vi "Sondenmodell.ReadZustandsgrössen.vi"(0 "Sondenmodell in":refnum<data-value>, 5 "error in":errorcluster) -> (14 "Sondenmodell out":refnum<data-value>, 16 "Erdtemperatur [°C]":dbl, 17 "Rücklauftemperatur Solekreislauf [°C]":dbl, 19 "error out":errorcluster)   [LabVIEW 2016, in "Sondenmodell.lvclass"]
uses:
  Sondenmodell.lvclass
  Sondenmodell.lvclass/Sondenmodell.ctl
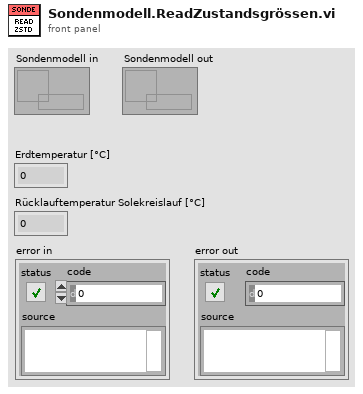
[diagram p1: front panel]
types:
  T1 = typedef "Sondenmodell.lvclass/Sondenmodell.Zustandsgrössen.ctl" = cluster{"Erdtemperatur [°C]":dbl, "Rücklauftemperatur Solekreislauf [°C]":dbl}
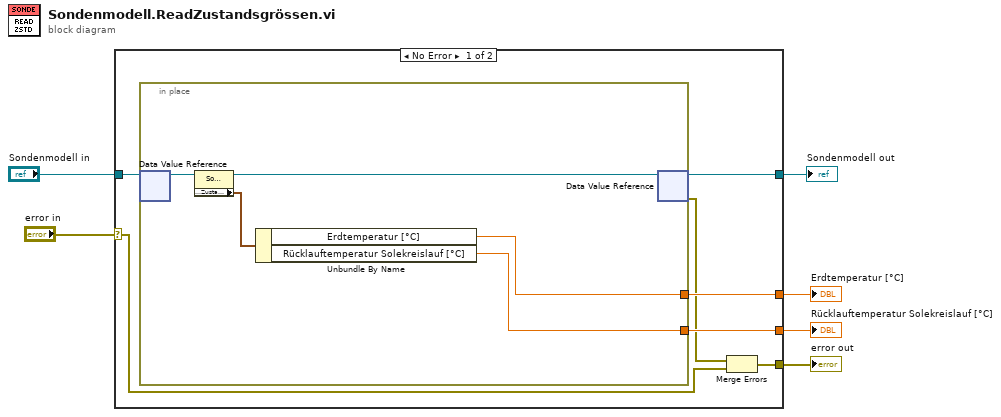
[diagram p0: block diagram]
diagram:
  n1 = case shown="No Error" "error in" {
    selector: "error in" -> [w8 w19]
    tunnel: [w13 w20] -> w6
    tunnel: [w12 _] -> w5
    tunnel: [w11 _] -> w4
    tunnel: "Sondenmodell in" -> [w10 w20]
    tunnel: [w7 w19] -> w1
    frame No Error {
      n2 = in-place {
        in-place-border: [w16] -> w12
        in-place-border: [w15] -> w11
        n3 = in-place-dvr #1(w10) -> (w18:refnum<class "Sondenmodell.lvclass">)  [unwired: 1 out]
        n4 = property class="Sondenmodell.lvclass"(reference=w18) -> (reference out=w17:refnum<class "Sondenmodell.lvclass">, "Accessors:Sondenmodell.Zustandsgrössen"=w14:T1)  [unwired: 1 in, 1 out]
        n5 = Unbundle By Name(w14) -> ("Erdtemperatur [°C]"=w16:dbl, "Rücklauftemperatur Solekreislauf [°C]"=w15:dbl)
        n6 = in-place-dvr #1(w17) -> (w13:refnum<data-value>, w9:errorcluster)
      }
      n7 = Merge Errors(w9, w8) -> (w7:errorcluster)
    }
    frame Error {
    }
  }
  "Erdtemperatur [°C]" <- w5
  "Rücklauftemperatur Solekreislauf [°C]" <- w4
  "Sondenmodell out" <- w6
  "error out" <- w1
